vi "joe_johnson.vi"() -> ()   [LabVIEW 2011]
uses:
  joe_johnson_state.ctl
  idg_trust_t.ctl
  <vilib>/Rock Robotics/WPI/Joystick/WPI_JoystickAxis.ctl
  <vilib>/Rock Robotics/WPI/Joystick/WPI_JoystickDevRef.ctl
  <vilib>/Rock Robotics/WPI/Joystick/WPI_JoystickDeviceEnum.ctl
  signals/Signal.ctl
  peg_leg_state.ctl
panel:
  in  "Ignore Limits":bool=TRUE
  in  "Peg High Limit":dbl=3.9
  in  "Peg Low Limit":dbl=2.5
  out "Voltage":dbl
  in  "Inverted":bool=TRUE
  out "error out 2":errorcluster
  out "Delta":dbl
  out "Integrator":u32
  # "Joe Johnson and Peg Leg controllers"
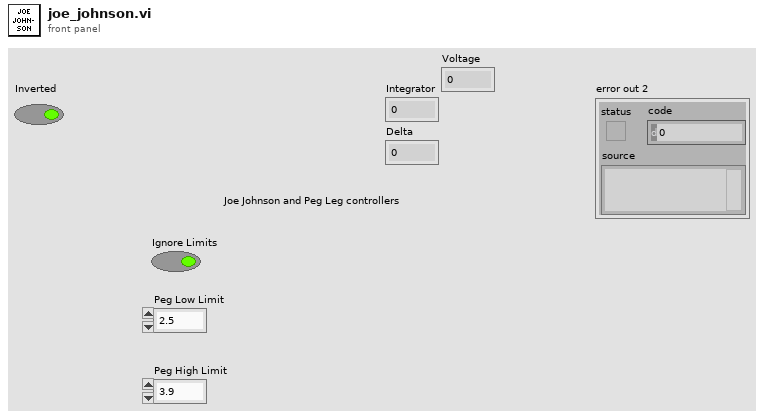
[diagram p1: front panel]
types:
  T1 = typedef "WPI_AnalogChannelDevRef.ctl" = cluster{"DevStatus":errorcluster, "Analog Module":T2, "Analog Channel":T3}
  T2 = typedef "FPGA_TypedefAnalogModule.ctl" = enum16{"Analog Module 1", "Analog Module 2"}
  T3 = typedef "FPGA_AIChannel.ctl" = enum8{"AI 1", "AI 2", "AI 3", "AI 4", "AI 5", "AI 6", "AI 7", "AI 8", "Invalid"}
  T4 = typedef "WPI_MotorControlDeviceRef.ctl" = cluster{"DeviceStatus":errorcluster, "Type":enum16{"PWM", "CAN"}, "PWM":cluster{"Digital Module":T5, "PWM Channel":T6, "DeadBand":T7}, "CAN":cluster{"Device Number":u8, "Control Mode":T8, "Semaphore":T9, "Max Vout":dbl}, "Invert":bool, "TransformRef":T10, "InvTransformRef":T10}
  T5 = typedef "FPGA_TypedefDigitalModule.ctl" = enum16{"Digital Module 1", "Digital Module 2"}
  T6 = typedef "FPGA_DIOPWMChannel.ctl" = enum8{"PWM 1", "PWM 2", "PWM 3", "PWM 4", "PWM 5", "PWM 6", "PWM 7", "PWM 8", "PWM 9", "PWM 10", "Invalid"}
  T7 = typedef "WPI_PWMDeadband.ctl" = cluster{"Name":string, "maxPositivePwm":i32, "minPositivePwm":i32, "centerPwm":i32, "maxNegativePwm":i32, "minNegativePwm":i32, "angularRange":u16}
  T8 = typedef "WPI_CANJaguar_ControlMode.ctl" = enum8{"Percent VBus", "Current", "Speed", "Position", "Voltage"}
  T9 = typedef "Semaphore RefNum" = refnum<k1>
  T10 = typedef "WPI_PWMTransform_ConPane.ctl" = refnum<vi>
  T11 = typedef "joe_johnson_state.ctl" = enum16{"fold", "down", "up", "ramp", "bridge_lift", "manual", "ramp_stay"}
  T12 = typedef "idg_trust_t.ctl" = enum16{"fault_move", "fault_high", "fault_low", "out_high", "out_low", "trust"}
  T13 = cluster{"analog":dbl, "input":dbl, "joe_johnson_state":T11, "idg_state":T12}
  T14 = enum16{"push_data", "write_joe_johnson", "write_roller", "write_drivetrain", "write_gun_fast", "write_gun_slow"}
  T15 = typedef "WPI_JoystickAxis.ctl" = enum16{"Axis 1", "Axis 2", "Axis 3", "Axis 4", "Axis 5", "Axis 6"}
  T16 = typedef "WPI_JoystickDevRef.ctl" = cluster{"Device":T17}
  T17 = typedef "WPI_JoystickDeviceEnum.ctl" = enum16{"USB 1", "USB 2", "USB 3", "USB 4", "Kinect 1", "Kinect 2"}
  T18 = typedef "Signal.ctl" = enum16{"SIGFIRE", "SIGSTOPSCRIPT", "SIGSTARTGUN", "SIGSTOPGUN", "SIGDISABLED", "SIGENABLED", "SIGUDPTIMEOUT", "SIGNEWVISION_REMOTE", "SIGNEWVISION_LOCAL", "SIGSHOTFIRED", "SIGDOTRACK", "SIGDONTTRACK"}
  T19 = typedef "peg_leg_state.ctl" = enum16{"up", "down", "unfold", "manual"}
  T20 = typedef "joe_johnson_const_t.ctl" = cluster{"joe_johnson":cluster{"joe_johnson_scale":T21, "joe_johnson_idg":T22, "joe_min_power":dbl, "joe_motor_invert":bool, "gain_scheduler":T23, "max_integral":dbl}}
  T21 = typedef "scale_const.ctl" = cluster{"min_ana":dbl, "min_units":dbl, "max_ana":dbl, "max_units":dbl}
  T22 = typedef "gun_idg_const.ctl" = cluster{"low_fault_ana":dbl, "high_fault_ana":dbl, "min_ana":dbl, "max_ana":dbl, "movement_thresh":dbl, "movement_time":dbl}
  T23 = typedef "gain_sched_const.ctl" = cluster{"pid_min":T24, "pid_max":T24, "min":dbl, "max":dbl}
  T24 = typedef "gain_const.ctl" = cluster{"kP":dbl, "kI":dbl, "kD":dbl}
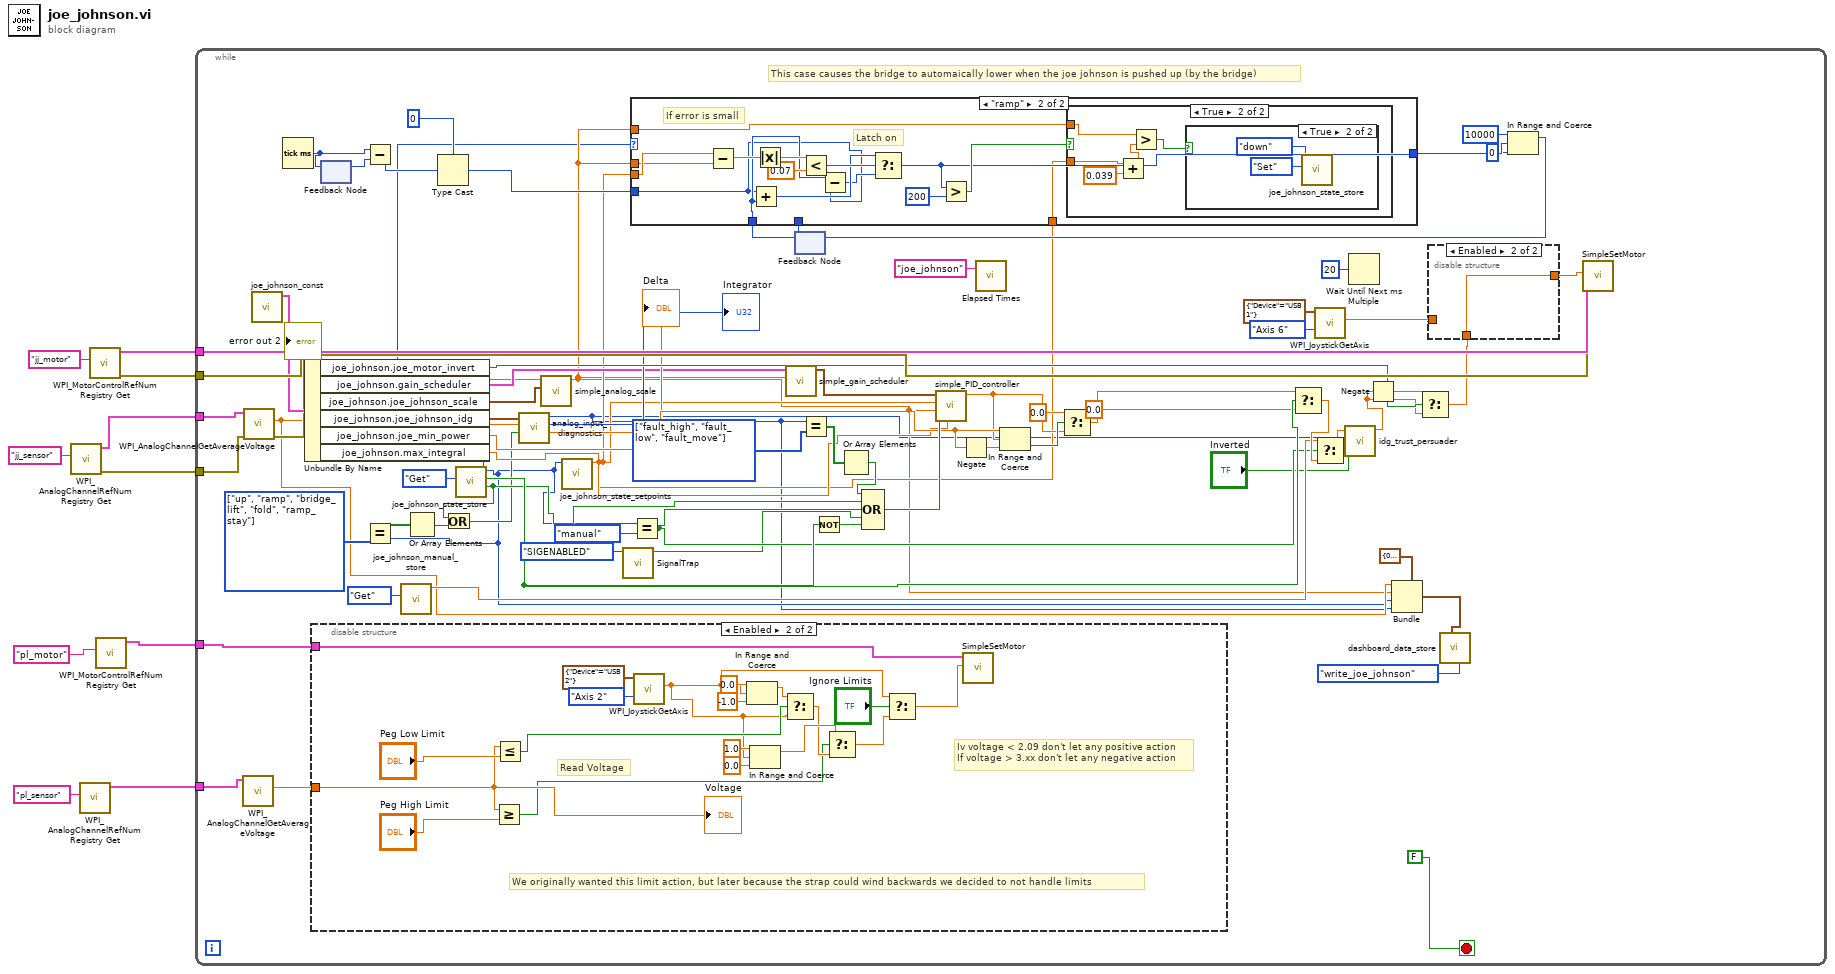
[diagram p0: block diagram]
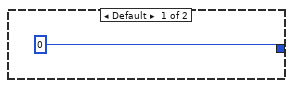
[diagram p3: hidden frame]
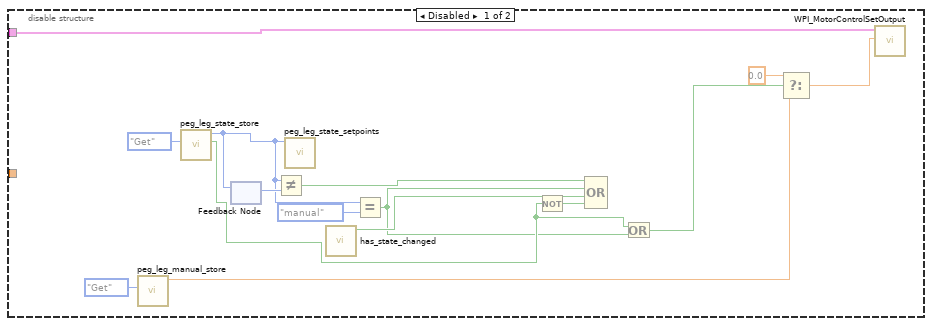
[diagram p6: hidden frame]
diagram:
  n1 = call <vilib>:"WPI_AnalogChannelRefNum Registry Get.vi"("refnum name"="jj_sensor") -> ("error out"=w4:errorcluster, "AIDeviceRef"=w6:T1)  [unwired: 9 in]
  n2 = call <vilib>:"WPI_AnalogChannelRefNum Registry Get.vi"("refnum name"="pl_sensor") -> ("AIDeviceRef"=w1:T1)  [unwired: 9 in, 1 out]
  n3 = call <vilib>:"WPI_MotorControlRefNum Registry Get.vi"("refnum name"="jj_motor") -> ("error out"=w3:errorcluster, "MotorControlDevRef"=w5:T4)  [unwired: 9 in]
  n4 = call <vilib>:"WPI_MotorControlRefNum Registry Get.vi"("refnum name"="pl_motor") -> ("MotorControlDevRef"=w7:T4)  [unwired: 9 in, 1 out]
  n5 = while {
    tunnel: w7 -> [w83]
    tunnel: w6 -> [w82]
    tunnel: w5 -> [w81]
    tunnel: w4 -> [w80]
    tunnel: w3 -> [w79]
    tunnel: w1 -> [w25]
    stop <- FALSE stop-if-true
    w57 = T11[] [enum."up", enum."ramp", enum."bridge_lift", enum."fold", enum."ramp_stay"] items=["fold", "down", "up", "ramp", "bridge_lift", "manual", "ramp_stay"]
    w74 = T12[] [enum."fault_high", enum."fault_low", enum."fault_move"] items=["fault_move", "fault_high", "fault_low", "out_high", "out_low", "trust"]
    # "This case causes the bridge to automaically lower when the joe johnson is pushed up (by the bridge)"
    n6 = call <vilib>:"WPI_AnalogChannelGetAverageVoltage.vi"("AIDeviceRef"=w25) -> ("Voltage"=w24:dbl)  [unwired: 8 in, 2 out]
    n7 = call <vilib>:"WPI_AnalogChannelGetAverageVoltage.vi"("error in (no error)"=w80, "AIDeviceRef"=w82) -> ("error out"=→"error out 2":errorcluster, "Voltage"=w14:dbl)  [unwired: 7 in, 1 out]
    n8 = call "joe_johnson_const.vi"() -> ("joe_johnson_const out"=w70:T20)  [unwired: 11 in]
    n9 = Tick Count (ms)() -> (millisecond timer value=w36:u32)
    n10 = Unbundle By Name(w70) -> ("joe_johnson.joe_motor_invert"=w62:bool, "joe_johnson.gain_scheduler"=w55:T23, "joe_johnson.joe_johnson_scale"=w78:T21, "joe_johnson.joe_johnson_idg"=w77:T22, "joe_johnson.joe_min_power"=w67:dbl, "joe_johnson.max_integral"=w49:dbl)
    n11 = disable-structure shown="Enabled" {
      disable-tunnel: w83 -> [w123 w142]
      disable-tunnel: w24 -> [_ w138]
      frame Disabled {
        n12 = call "peg_leg_manual_store.vi"("data_store_mode"=enum16{"Set", "Get"}."Get") -> ("Man Command Out"=w113:dbl)  [unwired: 10 in]
        n13 = call "peg_leg_state_store.vi"("data_store_mode"=enum16{"Set", "Get"}."Get") -> ("Initialized"=w112:bool, "peg_leg_state out"=w117:T19)  [unwired: 9 in]
        n14 = feedback #1() -> (w118:T19)  [unwired: 1 in]
        n15 = feedback-in #1(w117) -> ()
        n16 = Not Equal?(x=w117, y=w118) -> (x != y?=w121:bool)
        n17 = call "peg_leg_state_setpoints.vi"("peg_leg_state"=w117) -> ()  [unwired: 10 in, 1 out]
        n18 = call "has_state_changed.vi"() -> ("Just Enabled"=w120:bool)  [unwired: 8 in, 3 out]
        n19 = Equal?(x=w117, y=peg_leg_state."manual") -> (x = y?=w110:bool)
        n20 = Not(x=w112) -> (.not. x?=w119:bool)
        n21 = Compound Arithmetic op=OR(w121, w110, w120, w119) -> ()  [unwired: 1 out]
        n22 = Or(x=w112, y=w110) -> (x .or. y?=w111:bool)
        n23 = Select(t=0.0, s=w111, f=w113) -> (s? t:f=w115:dbl)
        n24 = call <vilib>:"WPI_MotorControlSetOutput.vi"("Output"=w115, "MotorControlDevRef"=w123) -> ()  [unwired: 8 in, 2 out]
      }
      frame Enabled {
        # "We originally wanted this limit action, but later because the strap could wind backwards we decided to not handle limits"
        # "Iv voltage < 2.09 don't let any positive action\nIf voltage > 3.xx don't let any negative action"
        # "Read Voltage"
        n25 = Greater Or Equal?(x=w138, y="Peg High Limit") -> (x >= y?=w128:bool)
        n26 = Less Or Equal?(x=w138, y="Peg Low Limit") -> (x <= y?=w129:bool)
        n27 = call <vilib>:"WPI_JoystickGetAxis.vi"("Axis"=WPI_JoystickAxis."Axis 2", "JoystickDevRef"=T16 {"Device"=enum."USB 2"}) -> ("Value"=w125:dbl)  [unwired: 8 in, 1 out]
        n28 = In Range and Coerce(upper limit=0.0, x=w125, lower limit=-1.0) -> (coerced(x)=w132:dbl)  [unwired: 1 out]
        n29 = In Range and Coerce(upper limit=1.0, x=w125, lower limit=0.0) -> (coerced(x)=w131:dbl)  [unwired: 1 out]
        n30 = Select(t=w132, s=w129, f=w125) -> (s? t:f=w130:dbl)
        n31 = Select(t=w131, s=w128, f=w130) -> (s? t:f=w127:dbl)
        n32 = Select(t=w125, s="Ignore Limits", f=w127) -> (s? t:f=w126:dbl)
        n33 = call "SimpleSetMotor.vi"("Output"=w126, "MotorControlDevRef"=w142) -> ()  [unwired: 8 in, 2 out]
        "Voltage" <- w138
      }
    }
    n34 = feedback-in #2(w36) -> ()
    n35 = feedback #2() -> (w35:u32)  [unwired: 1 in]
    n36 = Subtract(x=w36, y=w35) -> (x-y=w33:u32)
    n37 = call "joe_johnson_manual_store.vi"("data_store_mode"=enum16{"Set", "Get"}."Get") -> ("Man Command Out"=w45:dbl)  [unwired: 10 in]
    n38 = Type Cast(type=0, x=w33) -> (*(type *) &x=w31:i32)
    n39 = call "joe_johnson_state_store.vi"("data_store_mode"=enum16{"Set", "Get"}."Get") -> ("New Data"=w41:bool, "Initialized"=w48:bool, "joe_johnson_state out"=w12:T11)  [unwired: 8 in]
    n40 = Equal?(x=w57, y=w12) -> (x = y?=w56:bool[])
    n41 = Or Array Elements(Boolean array=w56) -> (logical OR=w40:bool)
    n42 = Or(x=w41, y=w40) -> (x .or. y?=w39:bool)
    n43 = call "analog_input_diagnostics.vi"("Reset Move Fault"=w39, "Voltage"=w14, "IDG Const"=w77) -> ("Delta"=→"Delta":dbl, "Integrator"=→"Integrator":u32, "IDG State"=w11:T12)  [unwired: 6 in]
    n44 = call "simple_analog_scale.vi"("Scale Const"=w78, "Analog"=w14) -> ("Units"=w13:dbl)  [unwired: 9 in]
    n45 = call "joe_johnson_state_setpoints.vi"("joe_johnson_state"=w12) -> ("setpoint"=w23:dbl)  [unwired: 10 in]
    n46 = call "SignalTrap.vi"("Signal"=Signal."SIGENABLED") -> ("Trapped Signal"=w43:bool)  [unwired: 10 in]
    n47 = Equal?(x=w12, y=joe_johnson_state."manual") -> (x = y?=w44:bool)
    n48 = call "simple_gain_scheduler.vi"("Scheduled Variable"=w13, "gain_scheduler"=w55) -> ("Gain"=w51:T24)  [unwired: 9 in]
    n49 = feedback #3() -> (w34:i32)  [unwired: 1 in]
    n50 = case shown="\"ramp\"" w12 {
      tunnel: w23 -> [_ w101]
      tunnel: w13 -> [_ w100]
      tunnel: w34 -> [_ _]
      tunnel: w13 -> [_ w95]
      tunnel: w31 -> [_ w89]
      tunnel: w34 -> [_ w90]
      tunnel: [0 w88] -> w30
      tunnel: w23 -> [_ w87]
      frame Default {
      }
      frame "ramp" {
        # "Latch on"
        # "If error is small"
        n51 = Subtract(x=w101, y=w100) -> (x-y=w99:dbl)
        n52 = Add(x=w89, y=w90) -> (x+y=w94:i32)
        n53 = Absolute Value(x=w99) -> (abs(x)=w98:dbl)
        n54 = Less?(x=w98, y=0.07) -> (x < y?=w96:bool)
        n55 = Subtract(x=w90, y=w89) -> (x-y=w91:i32)
        n56 = Select(t=w94, s=w96, f=w91) -> (s? t:f=w88:i32)
        n57 = Greater?(x=w88, y=200) -> (0:w93:bool)
        n58 = case shown="True" w93 {
          tunnel: w95 -> [_ w106]
          tunnel: w87 -> [_ w102]
          frame False {
          }
          frame True {
            n59 = Add(x=w102, y=0.039) -> (x+y=w103:dbl)
            n60 = Greater?(x=w106, y=w103) -> (0:w105:bool)
            n61 = case shown="True" w105 {
              frame False {
              }
              frame True {
                n62 = call "joe_johnson_state_store.vi"("data_store_mode"=enum16{"Set", "Get"}."Set", "joe_johnson_state"=joe_johnson_state."down") -> ()  [unwired: 7 in, 3 out]
              }
            }
          }
        }
      }
    }
    n63 = Equal?(x=w11, y=w74) -> (x = y?=w73:bool[])
    n64 = Not(x=w48) -> (.not. x?=w71:bool)
    n65 = Or Array Elements(Boolean array=w73) -> (logical OR=w72:bool)
    n66 = Compound Arithmetic op=OR(w72, w41, w44, w43, w71) -> (w76:bool)
    n67 = call "simple_PID_controller.vi"("Max Integral"=w49, "Reset Integral"=w76, "Sensor"=w13, "Setpoint"=w23, "PID Const"=w51) -> ("Motor Power"=w65:dbl)  [unwired: 6 in]
    n68 = Negate(x=w67) -> (-x=w68:dbl)
    n69 = call "Elapsed Times.vi"("Call Name"="joe_johnson") -> ()  [unwired: 2 in, 1 out]
    n70 = In Range and Coerce(upper limit=w67, x=w65, lower limit=w68) -> (In Range?=w66:bool)  [unwired: 1 out]
    n71 = Select(t=0.0, s=w66, f=w65) -> (s? t:f=w64:dbl)
    n72 = Select(t=w64, s=w48, f=0.0) -> (s? t:f=w46:dbl)
    n73 = call <vilib>:"WPI_JoystickGetAxis.vi"("Axis"=WPI_JoystickAxis."Axis 6", "JoystickDevRef"=T16 {"Device"=enum."USB 1"}) -> ("Value"=w18:dbl)  [unwired: 8 in, 1 out]
    n74 = Select(t=w45, s=w44, f=w46) -> (s? t:f=w38:dbl)
    n75 = call "idg_trust_persuader.vi"("Inverted"="Inverted", "Input Diagnostic State"=w11, "output"=w38) -> ("output out"=w37:dbl)  [unwired: 8 in]
    n76 = Wait Until Next ms Multiple(millisecond multiple=u32 20) -> ()  [unwired: 1 out]
    n77 = Negate(x=w37) -> (-x=w61:dbl)
    n78 = Bundle(cluster=T13 {"analog"=0.0, "input"=0.0, "joe_johnson_state"=enum."fold", "idg_state"=enum."fault_high"} ("joe_johnson_data"), "analog"=w14, "input"=w13, "joe_johnson_state"=w12, "idg_state"=w11) -> (w15:T13)
    n79 = Select(t=w61, s=w62, f=w37) -> (s? t:f=w22:dbl)
    n80 = disable-structure shown="Enabled" {
      disable-tunnel: w22 -> [_ w85]
      disable-tunnel: [w84 w85] -> w21
      disable-tunnel: w18 -> [w84 _]
      frame Disabled {
      }
      frame Enabled {
      }
    }
    n81 = call "dashboard_data_store.vi"("mode"=T14."write_joe_johnson", "joe_johnson_data"=w15) -> ()  [unwired: 10 in]
    n82 = In Range and Coerce(upper limit=10000, x=w30, lower limit=0) -> (coerced(x)=w27:i32)  [unwired: 1 out]
    n83 = feedback-in #3(w27) -> ()
    n84 = call "SimpleSetMotor.vi"("error in (no error)"=w79, "Output"=w21, "MotorControlDevRef"=w81) -> ()  [unwired: 7 in, 2 out]
  }
